vi "Lab Panel V5.31.vi"() -> ()   [LabVIEW 2017] (continued)
                            n2531 = Build Array(w4626) -> (w4623:dbl[])
                            n2532 = Build Array(w4631) -> (w4618:dbl[])
                            n2533 = Build Array("AMPS ON", "AMPS OFF", "VOLTS", "PF", "TEMP Live", "TEMP Neut", "CYCLE") -> (w4601:string[])
                            n2534 = Bundle By Name("Y"=w4624, "t0"=w4617) -> (w4616:waveform(dbl))  [unwired: 1 in]
                            n2535 = Bundle By Name("Y"=w4623, "t0"=w4617) -> (w4615:waveform(dbl))  [unwired: 1 in]
                            n2536 = Bundle By Name("Y"=w4622, "t0"=w4617) -> (w4614:waveform(dbl))  [unwired: 1 in]
                            n2537 = Bundle By Name("Y"=w4621, "t0"=w4617) -> (w4613:waveform(dbl))  [unwired: 1 in]
                            n2538 = Bundle By Name("Y"=w4620, "t0"=w4617) -> (w4612:waveform(dbl))  [unwired: 1 in]
                            n2539 = Bundle By Name("Y"=w4619, "t0"=w4617) -> (w4611:waveform(dbl))  [unwired: 1 in]
                            n2540 = Bundle By Name("Y"=w4618, "t0"=w4617) -> (w4610:waveform(dbl))  [unwired: 1 in]
                            n2541 = Build Array(w4616, w4615, w4614, w4613, w4612, w4611, w4610) -> (w4609:waveform(dbl)[])
                            n2542 = TDMS Write(0:w4630, 5:"TEST VALUES", 7:w4601, 9:w4609) -> (4:w4600:refnum<k34>, 6:w4599:string, 15:w4598:errorcluster)  [unwired: 2 in, 1 out]
                            n2543 = TDMS Write(0:w4600, 5:w4599, 7:"TIME", 9:w4596, 11:w4598) -> (15:w4595:errorcluster)  [unwired: 1 in, 3 out]
                            n2544 = local write "data file error"(w4595) -> ()
                          }
                        }
                      }
                    }
                  }
                }
              }
              frame #8 {
                n2545 = case shown="True" w4634 {
                  tunnel: w4638 -> [_ w4643]
                  tunnel: w4637 -> [_ w4642]
                  tunnel: w4636 -> [_ w4640]
                  tunnel: w4635 -> [_ w4639]
                  frame False {
                  }
                  frame True {
                    n2546 = local read "DISP LAB05-1"() -> (w4644:T4)
                    n2547 = local read "SIG LAB05-1"() -> (w4645:T2)
                    n2548 = local read "ON L05-1"() -> (w4641:cluster{"amps":dbl, "volts":dbl, "pf":dbl})
                    n2549 = Unbundle(w4645) -> ("AMPS"=w4651:dbl, "VOLTS"=w4649:dbl, "PF"=w4648:dbl, "Tmp Live"=w4647:dbl, "Tmp Neut"=w4650:dbl)
                    n2550 = Unbundle(w4644) -> ("CYCLE"=w4646:dbl)  [unwired: 2 out]
                    n2551 = stacked-sequence {
                      tunnel: w4651 -> [w4655 w4674]
                      tunnel: w4650 -> [_ w4673]
                      tunnel: w4649 -> [w4654 w4672]
                      tunnel: w4648 -> [w4653 w4671]
                      tunnel: w4647 -> [_ w4670]
                      tunnel: w4646 -> [_ w4669]
                      tunnel: w4643 -> [_ w4668]
                      tunnel: w4642 -> [w4656 _]
                      tunnel: w4641 -> [w4652 w4666]
                      tunnel: w4640 -> [_ w4667]
                      tunnel: w4639 -> [_ w4662]
                      frame #0 {
                        n2552 = case shown="True" w4656 {
                          tunnel: w4655 -> [_ w4661]
                          tunnel: w4654 -> [_ w4660]
                          tunnel: w4653 -> [_ w4659]
                          tunnel: w4652 -> [_ w4657]
                          frame False {
                          }
                          frame True {
                            n2553 = Bundle(cluster=w4657, "amps"=w4661, "volts"=w4660, "pf"=w4659) -> (w4658:cluster{"amps":dbl, "volts":dbl, "pf":dbl})
                            n2554 = local write "ON L05-1"(w4658) -> ()
                          }
                        }
                      }
                      frame #1 {
                        n2555 = Unbundle(w4666) -> ("amps"=w4665:dbl, "volts"=w4664:dbl, "pf"=w4663:dbl)
                        n2556 = case shown="True" w4667 {
                          tunnel: w4674 -> [_ w4706]
                          tunnel: w4673 -> [_ w4713]
                          tunnel: w4672 -> [_ _]
                          tunnel: w4671 -> [_ _]
                          tunnel: w4670 -> [_ w4712]
                          tunnel: w4669 -> [_ w4711]
                          tunnel: w4668 -> [_ w4676]
                          tunnel: w4665 -> [_ w4708]
                          tunnel: w4664 -> [_ w4707]
                          tunnel: w4663 -> [_ w4705]
                          tunnel: w4662 -> [_ w4697]
                          frame False {
                          }
                          frame True {
                            n2557 = local read "TDMS LAB05-1"() -> (w4710:refnum<k34>)
                            n2558 = Build Array(w4707) -> (w4702:dbl[])
                            n2559 = Build Array(w4705) -> (w4701:dbl[])
                            n2560 = Build Array(w4712) -> (w4700:dbl[])
                            n2561 = Build Array(w4713) -> (w4699:dbl[])
                            n2562 = Build Array(w4708) -> (w4704:dbl[])
                            n2563 = Build Array(w4706) -> (w4703:dbl[])
                            n2564 = Build Array(w4711) -> (w4698:dbl[])
                            n2565 = Build Array("AMPS ON", "AMPS OFF", "VOLTS", "PF", "TEMP Live", "TEMP Neut", "CYCLE") -> (w4681:string[])
                            n2566 = Bundle By Name("Y"=w4704, "t0"=w4697) -> (w4696:waveform(dbl))  [unwired: 1 in]
                            n2567 = Bundle By Name("Y"=w4703, "t0"=w4697) -> (w4695:waveform(dbl))  [unwired: 1 in]
                            n2568 = Bundle By Name("Y"=w4702, "t0"=w4697) -> (w4694:waveform(dbl))  [unwired: 1 in]
                            n2569 = Bundle By Name("Y"=w4701, "t0"=w4697) -> (w4693:waveform(dbl))  [unwired: 1 in]
                            n2570 = Bundle By Name("Y"=w4700, "t0"=w4697) -> (w4692:waveform(dbl))  [unwired: 1 in]
                            n2571 = Bundle By Name("Y"=w4699, "t0"=w4697) -> (w4691:waveform(dbl))  [unwired: 1 in]
                            n2572 = Bundle By Name("Y"=w4698, "t0"=w4697) -> (w4690:waveform(dbl))  [unwired: 1 in]
                            n2573 = Build Array(w4696, w4695, w4694, w4693, w4692, w4691, w4690) -> (w4689:waveform(dbl)[])
                            n2574 = TDMS Write(0:w4710, 5:"TEST VALUES", 7:w4681, 9:w4689) -> (4:w4680:refnum<k34>, 6:w4679:string, 15:w4678:errorcluster)  [unwired: 2 in, 1 out]
                            n2575 = TDMS Write(0:w4680, 5:w4679, 7:"TIME", 9:w4676, 11:w4678) -> (15:w4675:errorcluster)  [unwired: 1 in, 3 out]
                            n2576 = local write "data file error"(w4675) -> ()
                          }
                        }
                      }
                    }
                  }
                }
              }
              frame #9 {
                n2577 = case shown="True" w4714 {
                  tunnel: w4718 -> [_ w4723]
                  tunnel: w4717 -> [_ w4722]
                  tunnel: w4716 -> [_ w4720]
                  tunnel: w4715 -> [_ w4719]
                  frame False {
                  }
                  frame True {
                    n2578 = local read "DISP LAB05-2"() -> (w4724:T4)
                    n2579 = local read "SIG LAB05-2"() -> (w4725:T2)
                    n2580 = local read "ON L05-2"() -> (w4721:cluster{"amps":dbl, "volts":dbl, "pf":dbl})
                    n2581 = Unbundle(w4725) -> ("AMPS"=w4731:dbl, "VOLTS"=w4729:dbl, "PF"=w4728:dbl, "Tmp Live"=w4727:dbl, "Tmp Neut"=w4730:dbl)
                    n2582 = Unbundle(w4724) -> ("CYCLE"=w4726:dbl)  [unwired: 2 out]
                    n2583 = stacked-sequence {
                      tunnel: w4731 -> [w4735 w4754]
                      tunnel: w4730 -> [_ w4753]
                      tunnel: w4729 -> [w4734 w4752]
                      tunnel: w4728 -> [w4733 w4751]
                      tunnel: w4727 -> [_ w4750]
                      tunnel: w4726 -> [_ w4749]
                      tunnel: w4723 -> [_ w4748]
                      tunnel: w4722 -> [w4736 _]
                      tunnel: w4721 -> [w4732 w4746]
                      tunnel: w4720 -> [_ w4747]
                      tunnel: w4719 -> [_ w4742]
                      frame #0 {
                        n2584 = case shown="True" w4736 {
                          tunnel: w4735 -> [_ w4741]
                          tunnel: w4734 -> [_ w4740]
                          tunnel: w4733 -> [_ w4739]
                          tunnel: w4732 -> [_ w4737]
                          frame False {
                          }
                          frame True {
                            n2585 = Bundle(cluster=w4737, "amps"=w4741, "volts"=w4740, "pf"=w4739) -> (w4738:cluster{"amps":dbl, "volts":dbl, "pf":dbl})
                            n2586 = local write "ON L05-2"(w4738) -> ()
                          }
                        }
                      }
                      frame #1 {
                        n2587 = Unbundle(w4746) -> ("amps"=w4745:dbl, "volts"=w4744:dbl, "pf"=w4743:dbl)
                        n2588 = case shown="True" w4747 {
                          tunnel: w4754 -> [_ w4786]
                          tunnel: w4753 -> [_ w4793]
                          tunnel: w4752 -> [_ _]
                          tunnel: w4751 -> [_ _]
                          tunnel: w4750 -> [_ w4792]
                          tunnel: w4749 -> [_ w4791]
                          tunnel: w4748 -> [_ w4756]
                          tunnel: w4745 -> [_ w4788]
                          tunnel: w4744 -> [_ w4787]
                          tunnel: w4743 -> [_ w4785]
                          tunnel: w4742 -> [_ w4777]
                          frame False {
                          }
                          frame True {
                            n2589 = local read "TDMS LAB05-2"() -> (w4790:refnum<k34>)
                            n2590 = Build Array(w4787) -> (w4782:dbl[])
                            n2591 = Build Array(w4785) -> (w4781:dbl[])
                            n2592 = Build Array(w4792) -> (w4780:dbl[])
                            n2593 = Build Array(w4793) -> (w4779:dbl[])
                            n2594 = Build Array(w4788) -> (w4784:dbl[])
                            n2595 = Build Array(w4786) -> (w4783:dbl[])
                            n2596 = Build Array(w4791) -> (w4778:dbl[])
                            n2597 = Build Array("AMPS ON", "AMPS OFF", "VOLTS", "PF", "TEMP Live", "TEMP Neut", "CYCLE") -> (w4761:string[])
                            n2598 = Bundle By Name("Y"=w4784, "t0"=w4777) -> (w4776:waveform(dbl))  [unwired: 1 in]
                            n2599 = Bundle By Name("Y"=w4783, "t0"=w4777) -> (w4775:waveform(dbl))  [unwired: 1 in]
                            n2600 = Bundle By Name("Y"=w4782, "t0"=w4777) -> (w4774:waveform(dbl))  [unwired: 1 in]
                            n2601 = Bundle By Name("Y"=w4781, "t0"=w4777) -> (w4773:waveform(dbl))  [unwired: 1 in]
                            n2602 = Bundle By Name("Y"=w4780, "t0"=w4777) -> (w4772:waveform(dbl))  [unwired: 1 in]
                            n2603 = Bundle By Name("Y"=w4779, "t0"=w4777) -> (w4771:waveform(dbl))  [unwired: 1 in]
                            n2604 = Bundle By Name("Y"=w4778, "t0"=w4777) -> (w4770:waveform(dbl))  [unwired: 1 in]
                            n2605 = Build Array(w4776, w4775, w4774, w4773, w4772, w4771, w4770) -> (w4769:waveform(dbl)[])
                            n2606 = TDMS Write(0:w4790, 5:"TEST VALUES", 7:w4761, 9:w4769) -> (4:w4760:refnum<k34>, 6:w4759:string, 15:w4758:errorcluster)  [unwired: 2 in, 1 out]
                            n2607 = TDMS Write(0:w4760, 5:w4759, 7:"TIME", 9:w4756, 11:w4758) -> (15:w4755:errorcluster)  [unwired: 1 in, 3 out]
                            n2608 = local write "data file error"(w4755) -> ()
                          }
                        }
                      }
                    }
                  }
                }
              }
            }
          }
          frame #15 {
            # "display test values on chart"
            n2609 = local read "jig cycle"() -> (w4798:dbl)
            n2610 = local read "on loops"() -> (w4800:dbl)
            n2611 = Add(x=w4800, y=4) -> (x+y=w4797:dbl)
            n2612 = Equal?(x=w4798, y=3) -> (x = y?=w4796:bool)
            n2613 = Equal?(x=w4798, y=w4797) -> (x = y?=w4795:bool)
            n2614 = Or(x=w4796, y=w4795) -> (x .or. y?=w4794:bool)
            "graph flag" <- w4794
            n2615 = global write "Global display 3.vi" "graph flag"(w4794) -> ()
            n2616 = case shown="True" w4794 {
              frame False {
              }
              frame True {
                n2617 = local read "SIG LAB05-1"() -> (w4843:T2)
                n2618 = local read "SIG LAB04-2"() -> (w4844:T2)
                n2619 = local read "SIG LAB05-2"() -> (w4842:T2)
                n2620 = local read "SIG LAB04-1"() -> (w4845:T2)
                n2621 = local read "SIG LAB01-1"() -> (w4851:T2)
                n2622 = local read "SIG LAB03-1"() -> (w4847:T2)
                n2623 = local read "SIG LAB03-2"() -> (w4846:T2)
                n2624 = local read "SIG LAB02-2"() -> (w4848:T2)
                n2625 = local read "SIG LAB02-1"() -> (w4849:T2)
                n2626 = local read "SIG LAB01-2"() -> (w4850:T2)
                n2627 = Unbundle By Name(w4851) -> ("AMPS"=w4841:dbl, "VOLTS"=w4831:dbl, "Tmp Live"=w4821:dbl, "Tmp Neut"=w4811:dbl)
                n2628 = Unbundle(w4844) -> ("AMPS"=w4834:dbl, "VOLTS"=w4824:dbl, "Tmp Live"=w4814:dbl, "Tmp Neut"=w4804:dbl)  [unwired: 1 out]
                n2629 = Unbundle(w4843) -> ("AMPS"=w4833:dbl, "VOLTS"=w4823:dbl, "Tmp Live"=w4813:dbl, "Tmp Neut"=w4803:dbl)  [unwired: 1 out]
                n2630 = Unbundle(w4842) -> ("AMPS"=w4832:dbl, "VOLTS"=w4822:dbl, "Tmp Live"=w4812:dbl, "Tmp Neut"=w4802:dbl)  [unwired: 1 out]
                n2631 = Unbundle(w4845) -> ("AMPS"=w4835:dbl, "VOLTS"=w4825:dbl, "Tmp Live"=w4815:dbl, "Tmp Neut"=w4805:dbl)  [unwired: 1 out]
                n2632 = Unbundle(w4846) -> ("AMPS"=w4836:dbl, "VOLTS"=w4826:dbl, "Tmp Live"=w4816:dbl, "Tmp Neut"=w4806:dbl)  [unwired: 1 out]
                n2633 = Unbundle(w4847) -> ("AMPS"=w4837:dbl, "VOLTS"=w4827:dbl, "Tmp Live"=w4817:dbl, "Tmp Neut"=w4807:dbl)  [unwired: 1 out]
                n2634 = Unbundle(w4848) -> ("AMPS"=w4838:dbl, "VOLTS"=w4828:dbl, "Tmp Live"=w4818:dbl, "Tmp Neut"=w4808:dbl)  [unwired: 1 out]
                n2635 = Unbundle(w4849) -> ("AMPS"=w4839:dbl, "VOLTS"=w4829:dbl, "Tmp Live"=w4819:dbl, "Tmp Neut"=w4809:dbl)  [unwired: 1 out]
                n2636 = Unbundle(w4850) -> ("AMPS"=w4840:dbl, "VOLTS"=w4830:dbl, "Tmp Live"=w4820:dbl, "Tmp Neut"=w4810:dbl)  [unwired: 1 out]
                n2637 = stacked-sequence {
                  tunnel: w4841 -> [w4883 _ _]
                  tunnel: w4840 -> [w4882 _ _]
                  tunnel: w4839 -> [w4873 _ _]
                  tunnel: w4838 -> [w4872 _ _]
                  tunnel: w4837 -> [w4862 _ _]
                  tunnel: w4836 -> [w4861 _ _]
                  tunnel: w4835 -> [_ w4906 _]
                  tunnel: w4834 -> [_ w4905 _]
                  tunnel: w4833 -> [_ w4895 _]
                  tunnel: w4832 -> [_ w4894 _]
                  tunnel: w4831 -> [w4880 _ _]
                  tunnel: w4830 -> [w4879 _ _]
                  tunnel: w4829 -> [w4870 _ _]
                  tunnel: w4828 -> [w4869 _ _]
                  tunnel: w4827 -> [w4860 _ _]
                  tunnel: w4826 -> [w4859 _ _]
                  tunnel: w4825 -> [_ w4904 _]
                  tunnel: w4824 -> [_ w4903 _]
                  tunnel: w4823 -> [_ w4893 _]
                  tunnel: w4822 -> [_ w4892 _]
                  tunnel: w4821 -> [w4877 _ _]
                  tunnel: w4820 -> [w4875 _ _]
                  tunnel: w4819 -> [w4866 _ _]
                  tunnel: w4818 -> [w4864 _ _]
                  tunnel: w4817 -> [w4858 _ _]
                  tunnel: w4816 -> [w4856 _ _]
                  tunnel: w4815 -> [_ w4902 _]
                  tunnel: w4814 -> [_ w4900 _]
                  tunnel: w4813 -> [_ w4891 _]
                  tunnel: w4812 -> [_ w4889 _]
                  tunnel: w4811 -> [w4876 _ _]
                  tunnel: w4810 -> [w4874 _ _]
                  tunnel: w4809 -> [w4865 _ _]
                  tunnel: w4808 -> [w4863 _ _]
                  tunnel: w4807 -> [w4857 _ _]
                  tunnel: w4806 -> [w4855 _ _]
                  tunnel: w4805 -> [_ w4901 _]
                  tunnel: w4804 -> [_ w4899 _]
                  tunnel: w4803 -> [_ w4890 _]
                  tunnel: w4802 -> [_ w4888 _]
                  frame #0 {
                    n2638 = Merge Signals(w4883, w4882) -> (→"LAB01 AMPS":dynamicdata)
                    n2639 = Merge Signals(w4880, w4879) -> (→"LAB01 VOLTS":dynamicdata)
                    n2640 = Merge Signals(w4860, w4859) -> (→"LAB03 VOLTS":dynamicdata)
                    n2641 = Merge Signals(w4877, w4876, w4875, w4874) -> (→"LAB01 deg C":dynamicdata)
                    n2642 = Merge Signals(w4873, w4872) -> (→"LAB02 AMPS":dynamicdata)
                    n2643 = Merge Signals(w4866, w4865, w4864, w4863) -> (→"LAB02 deg C":dynamicdata)
                    n2644 = Merge Signals(w4858, w4857, w4856, w4855) -> (→"LAB03 deg C":dynamicdata)
                    n2645 = Merge Signals(w4870, w4869) -> (→"LAB02 VOLTS":dynamicdata)
                    n2646 = Merge Signals(w4862, w4861) -> (→"LAB03 AMPS":dynamicdata)
                  }
                  frame #1 {
                    n2647 = Merge Signals(w4893, w4892) -> (→"LAB05 VOLTS":dynamicdata)
                    n2648 = Merge Signals(w4906, w4905) -> (→"LAB04 AMPS":dynamicdata)
                    n2649 = Merge Signals(w4895, w4894) -> (→"LAB05 AMPS":dynamicdata)
                    n2650 = Merge Signals(w4891, w4890, w4889, w4888) -> (→"LAB05 deg C":dynamicdata)
                    n2651 = Merge Signals(w4902, w4901, w4900, w4899) -> (→"LAB04 deg C":dynamicdata)
                    n2652 = Merge Signals(w4904, w4903) -> (→"LAB04 VOLTS":dynamicdata)
                  }
                  frame #2 {
                    n2653 = local read "LAB05 VOLTS"() -> (w4914:dynamicdata)
                    n2654 = local read "LAB04 VOLTS"() -> (w4915:dynamicdata)
                    n2655 = local read "LAB05 AMPS"() -> (w4920:dynamicdata)
                    n2656 = local read "LAB02 VOLTS"() -> (w4917:dynamicdata)
                    n2657 = local read "LAB03 VOLTS"() -> (w4916:dynamicdata)
                    n2658 = local read "LAB01 VOLTS"() -> (w4918:dynamicdata)
                    n2659 = local read "LAB04 AMPS"() -> (w4921:dynamicdata)
                    n2660 = local read "LAB03 AMPS"() -> (w4922:dynamicdata)
                    n2661 = local read "LAB03 deg C"() -> (w4910:dynamicdata)
                    n2662 = local read "LAB02 AMPS"() -> (w4923:dynamicdata)
                    n2663 = local read "LAB04 deg C"() -> (w4909:dynamicdata)
                    n2664 = local read "LAB05 deg C"() -> (w4908:dynamicdata)
                    n2665 = local read "LAB02 deg C"() -> (w4911:dynamicdata)
                    n2666 = local read "LAB01 deg C"() -> (w4912:dynamicdata)
                    n2667 = local read "LAB01 AMPS"() -> (w4924:dynamicdata)
                    n2668 = Merge Signals(w4912, w4911, w4910, w4909, w4908) -> (w4907:dynamicdata)
                    n2669 = Merge Signals(w4924, w4923, w4922, w4921, w4920) -> (w4919:dynamicdata)
                    n2670 = Merge Signals(w4918, w4917, w4916, w4915, w4914) -> (w4913:dynamicdata)
                    n2671 = global write "Global display 3.vi" "graph volts"(w4913) -> ()
                    n2672 = global write "Global display 3.vi" "graph deg C"(w4907) -> ()
                    n2673 = global write "Global display 3.vi" "graph amps"(w4919) -> ()
                  }
                }
              }
            }
          }
          frame #16 {
            # "check for amps fail"
            # "check for cycle test & temperature rise fail conditions"
            n2674 = local read "on loops"() -> (w4951:dbl)
            n2675 = local read "jig cycle"() -> (w4948:dbl)
            n2676 = Add(x=w4951, y=5.0) -> (x+y=w4949:dbl)
            n2677 = Equal?(x=w4948, y=w4949) -> (x = y?=w4944:bool)
            n2678 = local read "jig cycle"() -> (w4953:dbl)
            n2679 = Equal?(x=w4953, y=3.0) -> (x = y?=w4946:bool)
            n2680 = local read "Fail Loops"() -> (w4925:dbl)
            n2681 = stacked-sequence {
              tunnel: w4947 -> [w4956 _ _ _ _ _ _ _ _ _]
              tunnel: w4946 -> [w4957 w4977 w4997 w5017 w5037 w5057 w5077 w5097 w5117 w5137]
              tunnel: w4945 -> [w4954 _ _ _ _ _ _ _ _ _]
              tunnel: w4944 -> [w4955 w4976 w4996 w5016 w5036 w5056 w5076 w5096 w5116 w5136]
              tunnel: w4943 -> [_ w4975 _ _ _ _ _ _ _ _]
              tunnel: w4942 -> [_ w4974 _ _ _ _ _ _ _ _]
              tunnel: w4941 -> [_ _ w4995 _ _ _ _ _ _ _]
              tunnel: w4940 -> [_ _ w4994 _ _ _ _ _ _ _]
              tunnel: w4939 -> [_ _ _ w5015 _ _ _ _ _ _]
              tunnel: w4938 -> [_ _ _ w5014 _ _ _ _ _ _]
              tunnel: w4937 -> [_ _ _ _ w5035 _ _ _ _ _]
              tunnel: w4936 -> [_ _ _ _ w5034 _ _ _ _ _]
              tunnel: w4935 -> [_ _ _ _ _ w5055 _ _ _ _]
              tunnel: w4934 -> [_ _ _ _ _ w5054 _ _ _ _]
              tunnel: w4933 -> [_ _ _ _ _ _ w5075 _ _ _]
              tunnel: w4932 -> [_ _ _ _ _ _ w5074 _ _ _]
              tunnel: w4931 -> [_ _ _ _ _ _ _ w5095 _ _]
              tunnel: w4930 -> [_ _ _ _ _ _ _ w5094 _ _]
              tunnel: w4929 -> [_ _ _ _ _ _ _ _ w5115 _]
              tunnel: w4928 -> [_ _ _ _ _ _ _ _ w5114 _]
              tunnel: w4927 -> [_ _ _ _ _ _ _ _ _ w5135]
              tunnel: w4926 -> [_ _ _ _ _ _ _ _ _ w5134]
              frame #0 {
                # "LAB01-1"
                n2682 = case shown="True" w4954 {
                  tunnel: w4957 -> [_ w4970]
                  tunnel: w4956 -> [_ w4967]
                  tunnel: w4955 -> [_ w4966]
                  frame False {
                  }
                  frame True {
                    n2683 = local read "TEMP START LAB01-1"() -> (w4972:cluster{"TL":dbl, "TN":dbl})
                    n2684 = local read "RESULT LAB01-1"() -> (w4961:bool)
                    n2685 = local read "FAIL LAB01-1"() -> (w4964:cluster{"LO":dbl, "HI":dbl})
                    n2686 = local read "TDMS LAB01-1"() -> (w4971:refnum<k34>)
                    n2687 = local read "SET LAB01-1"() -> (w4968:T6)
                    n2688 = local read "DISP LAB01-1"() -> (w4969:T4)
                    n2689 = local read "SIG LAB01-1"() -> (w4973:T2)
                    n2690 = Bundle("FAIL LAB01-1"=w4964, "SIG LAB01-1"=w4973, "TEMP START LAB01-1"=w4972, "DISP LAB01-1"=w4969, "SET LAB01-1"=w4968, "TDMS LAB01-1"=w4971) -> (w4958:T36)  [unwired: 1 in]
                    n2691 = call "sub vi - cycle&temp fail v7.vi"("Amps Lo?"=w4970, "Input Cluster"=w4958, "SELECT"=w4967, "Amps Hi?"=w4966, "Result In"=w4961) -> ("(FAIL) out"=w4963:cluster{"FAIL LO":dbl, "FAIL HI":dbl}, "(DISP) out"=w4959:T4, "T-RISE"=w4960:cluster{"T-RISE (L)":dbl, "T-RISE (N)":dbl}, "Result Out"=w4962:bool, "file error"=w4965:errorcluster)  [unwired: 10 in]
                    n2692 = local write "TEMP RISE LAB01-1"(w4960) -> ()
                    n2693 = local write "FAIL LAB01-1"(w4963) -> ()
                    n2694 = local write "DISP LAB01-1"(w4959) -> ()
                    n2695 = local write "RESULT LAB01-1"(w4962) -> ()
                    n2696 = local write "data file error"(w4965) -> ()
                  }
                }
              }
              frame #1 {
                # "LAB01-2"
                n2697 = case shown="True" w4975 {
                  tunnel: w4977 -> [_ w4990]
                  tunnel: w4974 -> [_ w4987]
                  tunnel: w4976 -> [_ w4986]
                  frame False {
                  }
                  frame True {
                    n2698 = local read "TEMP START LAB01-2"() -> (w4992:cluster{"TL":dbl, "TN":dbl})
                    n2699 = local read "FAIL LAB01-2"() -> (w4983:cluster{"LO":dbl, "HI":dbl})
                    n2700 = local read "TDMS LAB01-2"() -> (w4991:refnum<k34>)
                    n2701 = local read "SET LAB01-2"() -> (w4988:T5)
                    n2702 = local read "DISP LAB01-2"() -> (w4989:T4)
                    n2703 = local read "RESULT LAB01-2"() -> (w4980:bool)
                    n2704 = local read "SIG LAB01-2"() -> (w4993:T2)
                    n2705 = Bundle("FAIL LAB01-2"=w4983, "SIG LAB01-2"=w4993, "TEMP START LAB01-2"=w4992, "DISP LAB01-2"=w4989, "SET LAB01-2"=w4988, "TDMS LAB01-2"=w4991) -> (w4978:T37)  [unwired: 1 in]
                    n2706 = call "sub vi - cycle&temp fail v7.vi"("Amps Lo?"=w4990, "Input Cluster"=w4978, "SELECT"=w4987, "Amps Hi?"=w4986, "Result In"=w4980) -> ("(FAIL) out"=w4982:cluster{"FAIL LO":dbl, "FAIL HI":dbl}, "(DISP) out"=w4985:T4, "T-RISE"=w4979:cluster{"T-RISE (L)":dbl, "T-RISE (N)":dbl}, "Result Out"=w4981:bool, "file error"=w4984:errorcluster)  [unwired: 10 in]
                    n2707 = local write "TEMP RISE LAB01-2"(w4979) -> ()
                    n2708 = local write "FAIL LAB01-2"(w4982) -> ()
                    n2709 = local write "DISP LAB01-2"(w4985) -> ()
                    n2710 = local write "RESULT LAB01-2"(w4981) -> ()
                    n2711 = local write "data file error"(w4984) -> ()
                  }
                }
              }
              frame #2 {
                # "LAB02-1"
                n2712 = case shown="True" w4995 {
                  tunnel: w4997 -> [_ w5010]
                  tunnel: w4994 -> [_ w5007]
                  tunnel: w4996 -> [_ w5006]
                  frame False {
                  }
                  frame True {
                    n2713 = local read "TEMP START LAB02-1"() -> (w5012:cluster{"TL":dbl, "TN":dbl})
                    n2714 = local read "FAIL LAB02-1"() -> (w5003:cluster{"LO":dbl, "HI":dbl})
                    n2715 = local read "TDMS LAB02-1"() -> (w5011:refnum<k34>)
                    n2716 = local read "SET LAB02-1"() -> (w5008:T5)
                    n2717 = local read "DISP LAB02-1"() -> (w5009:T4)
                    n2718 = local read "SIG LAB02-1"() -> (w5013:T2)
                    n2719 = local read "RESULT LAB02-1"() -> (w5000:bool)
                    n2720 = Bundle("FAIL LAB02-1"=w5003, "SIG LAB02-1"=w5013, "TEMP START LAB02-1"=w5012, "DISP LAB02-1"=w5009, "SET LAB02-1"=w5008, "TDMS LAB02-1"=w5011) -> (w4998:T38)  [unwired: 1 in]
                    n2721 = call "sub vi - cycle&temp fail v7.vi"("Amps Lo?"=w5010, "Input Cluster"=w4998, "SELECT"=w5007, "Amps Hi?"=w5006, "Result In"=w5000) -> ("(FAIL) out"=w5002:cluster{"FAIL LO":dbl, "FAIL HI":dbl}, "(DISP) out"=w5005:T4, "T-RISE"=w4999:cluster{"T-RISE (L)":dbl, "T-RISE (N)":dbl}, "Result Out"=w5001:bool, "file error"=w5004:errorcluster)  [unwired: 10 in]
                    n2722 = local write "TEMP RISE LAB02-1"(w4999) -> ()
                    n2723 = local write "FAIL LAB02-1"(w5002) -> ()
                    n2724 = local write "DISP LAB02-1"(w5005) -> ()
                    n2725 = local write "RESULT LAB02-1"(w5001) -> ()
                    n2726 = local write "data file error"(w5004) -> ()
                  }
                }
              }
              frame #3 {
                # "LAB02-2"
                n2727 = case shown="True" w5015 {
                  tunnel: w5017 -> [_ w5030]
                  tunnel: w5014 -> [_ w5027]
                  tunnel: w5016 -> [_ w5026]
                  frame False {
                  }
                  frame True {
                    n2728 = local read "TEMP START LAB02-2"() -> (w5032:cluster{"TL":dbl, "TN":dbl})
                    n2729 = local read "FAIL LAB02-2"() -> (w5023:cluster{"LO":dbl, "HI":dbl})
                    n2730 = local read "TDMS LAB02-2"() -> (w5031:refnum<k34>)
                    n2731 = local read "SET LAB02-2"() -> (w5028:T5)
                    n2732 = local read "DISP LAB02-2"() -> (w5029:T4)
                    n2733 = local read "SIG LAB02-2"() -> (w5033:T2)
                    n2734 = local read "RESULT LAB02-2"() -> (w5020:bool)
                    n2735 = Bundle("FAIL LAB02-2"=w5023, "SIG LAB02-2"=w5033, "TEMP START LAB02-2"=w5032, "DISP LAB02-2"=w5029, "SET LAB02-2"=w5028, "TDMS LAB02-2"=w5031) -> (w5018:T39)  [unwired: 1 in]
                    n2736 = call "sub vi - cycle&temp fail v7.vi"("Amps Lo?"=w5030, "Input Cluster"=w5018, "SELECT"=w5027, "Amps Hi?"=w5026, "Result In"=w5020) -> ("(FAIL) out"=w5022:cluster{"FAIL LO":dbl, "FAIL HI":dbl}, "(DISP) out"=w5025:T4, "T-RISE"=w5019:cluster{"T-RISE (L)":dbl, "T-RISE (N)":dbl}, "Result Out"=w5021:bool, "file error"=w5024:errorcluster)  [unwired: 10 in]
                    n2737 = local write "TEMP RISE LAB02-2"(w5019) -> ()
                    n2738 = local write "FAIL LAB02-2"(w5022) -> ()
                    n2739 = local write "DISP LAB02-2"(w5025) -> ()
                    n2740 = local write "RESULT LAB02-2"(w5021) -> ()
                    n2741 = local write "data file error"(w5024) -> ()
                  }
                }
              }
              frame #4 {
                # "LAB03-1"
                n2742 = case shown="True" w5035 {
                  tunnel: w5037 -> [_ w5050]
                  tunnel: w5034 -> [_ w5047]
                  tunnel: w5036 -> [_ w5046]
                  frame False {
                  }
                  frame True {
                    n2743 = local read "TEMP START LAB03-1"() -> (w5052:cluster{"TL":dbl, "TN":dbl})
                    n2744 = local read "FAIL LAB03-1"() -> (w5043:cluster{"LO":dbl, "HI":dbl})
                    n2745 = local read "TDMS LAB03-1"() -> (w5051:refnum<k34>)
                    n2746 = local read "SET LAB03-1"() -> (w5048:T5)
                    n2747 = local read "DISP LAB03-1"() -> (w5049:T4)
                    n2748 = local read "SIG LAB03-1"() -> (w5053:T2)
                    n2749 = local read "RESULT LAB03-1"() -> (w5040:bool)
                    n2750 = Bundle("FAIL LAB03-1"=w5043, "SIG LAB03-1"=w5053, "TEMP START LAB03-1"=w5052, "DISP LAB03-1"=w5049, "SET LAB03-1"=w5048, "TDMS LAB03-1"=w5051) -> (w5038:T40)  [unwired: 1 in]
                    n2751 = call "sub vi - cycle&temp fail v7.vi"("Amps Lo?"=w5050, "Input Cluster"=w5038, "SELECT"=w5047, "Amps Hi?"=w5046, "Result In"=w5040) -> ("(FAIL) out"=w5042:cluster{"FAIL LO":dbl, "FAIL HI":dbl}, "(DISP) out"=w5045:T4, "T-RISE"=w5039:cluster{"T-RISE (L)":dbl, "T-RISE (N)":dbl}, "Result Out"=w5041:bool, "file error"=w5044:errorcluster)  [unwired: 10 in]
                    n2752 = local write "TEMP RISE LAB03-1"(w5039) -> ()
                    n2753 = local write "FAIL LAB03-1"(w5042) -> ()
                    n2754 = local write "DISP LAB03-1"(w5045) -> ()
                    n2755 = local write "RESULT LAB03-1"(w5041) -> ()
                    n2756 = local write "data file error"(w5044) -> ()
                  }
                }
              }
              frame #5 {
                # "LAB03-2"
                n2757 = case shown="True" w5055 {
                  tunnel: w5057 -> [_ w5070]
                  tunnel: w5054 -> [_ w5067]
                  tunnel: w5056 -> [_ w5066]
                  frame False {
                  }
                  frame True {
                    n2758 = local read "TEMP START LAB03-2"() -> (w5072:cluster{"TL":dbl, "TN":dbl})
                    n2759 = local read "FAIL LAB03-2"() -> (w5063:cluster{"LO":dbl, "HI":dbl})
                    n2760 = local read "TDMS LAB03-2"() -> (w5071:refnum<k34>)
                    n2761 = local read "SET LAB03-2"() -> (w5068:T5)
                    n2762 = local read "DISP LAB03-2"() -> (w5069:T4)
                    n2763 = local read "RESULT LAB03-2"() -> (w5060:bool)
                    n2764 = local read "SIG LAB03-2"() -> (w5073:T2)
                    n2765 = Bundle("FAIL LAB03-2"=w5063, "SIG LAB03-2"=w5073, "TEMP START LAB03-2"=w5072, "DISP LAB03-2"=w5069, "SET LAB03-2"=w5068, "TDMS LAB03-2"=w5071) -> (w5058:T41)  [unwired: 1 in]
                    n2766 = call "sub vi - cycle&temp fail v7.vi"("Amps Lo?"=w5070, "Input Cluster"=w5058, "SELECT"=w5067, "Amps Hi?"=w5066, "Result In"=w5060) -> ("(FAIL) out"=w5062:cluster{"FAIL LO":dbl, "FAIL HI":dbl}, "(DISP) out"=w5065:T4, "T-RISE"=w5059:cluster{"T-RISE (L)":dbl, "T-RISE (N)":dbl}, "Result Out"=w5061:bool, "file error"=w5064:errorcluster)  [unwired: 10 in]
                    n2767 = local write "FAIL LAB03-2"(w5062) -> ()
                    n2768 = local write "TEMP RISE LAB03-2"(w5059) -> ()
                    n2769 = local write "DISP LAB03-2"(w5065) -> ()
                    n2770 = local write "RESULT LAB03-2"(w5061) -> ()
                    n2771 = local write "data file error"(w5064) -> ()
                  }
                }
              }
              frame #6 {
                # "LAB04-1"
                n2772 = case shown="True" w5075 {
                  tunnel: w5077 -> [_ w5090]
                  tunnel: w5074 -> [_ w5087]
                  tunnel: w5076 -> [_ w5086]
                  frame False {
                  }
                  frame True {
                    n2773 = local read "TEMP START LAB04-1"() -> (w5092:cluster{"TL":dbl, "TN":dbl})
                    n2774 = local read "FAIL LAB04-1"() -> (w5083:cluster{"LO":dbl, "HI":dbl})
                    n2775 = local read "TDMS LAB04-1"() -> (w5091:refnum<k34>)
                    n2776 = local read "SET LAB04-1"() -> (w5088:T5)
                    n2777 = local read "DISP LAB04-1"() -> (w5089:T4)
                    n2778 = local read "SIG LAB04-1"() -> (w5093:T2)
                    n2779 = local read "RESULT LAB04-1"() -> (w5080:bool)
                    n2780 = Bundle("FAIL LAB04-1"=w5083, "SIG LAB04-1"=w5093, "TEMP START LAB04-1"=w5092, "DISP LAB04-1"=w5089, "SET LAB04-1"=w5088, "TDMS LAB04-1"=w5091) -> (w5078:T42)  [unwired: 1 in]
                    n2781 = call "sub vi - cycle&temp fail v7.vi"("Amps Lo?"=w5090, "Input Cluster"=w5078, "SELECT"=w5087, "Amps Hi?"=w5086, "Result In"=w5080) -> ("(FAIL) out"=w5082:cluster{"FAIL LO":dbl, "FAIL HI":dbl}, "(DISP) out"=w5085:T4, "T-RISE"=w5079:cluster{"T-RISE (L)":dbl, "T-RISE (N)":dbl}, "Result Out"=w5081:bool, "file error"=w5084:errorcluster)  [unwired: 10 in]
                    n2782 = local write "TEMP RISE LAB04-1"(w5079) -> ()
                    n2783 = local write "FAIL LAB04-1"(w5082) -> ()
                    n2784 = local write "DISP LAB04-1"(w5085) -> ()
                    n2785 = local write "RESULT LAB04-1"(w5081) -> ()
                    n2786 = local write "data file error"(w5084) -> ()
                  }
                }
              }
              frame #7 {
                # "LAB04-2"
                n2787 = case shown="True" w5095 {
                  tunnel: w5097 -> [_ w5110]
                  tunnel: w5094 -> [_ w5107]
                  tunnel: w5096 -> [_ w5106]
                  frame False {
                  }
                  frame True {
                    n2788 = local read "TEMP START LAB04-2"() -> (w5112:cluster{"TL":dbl, "TN":dbl})
                    n2789 = local read "FAIL LAB04-2"() -> (w5103:cluster{"LO":dbl, "HI":dbl})
                    n2790 = local read "TDMS LAB04-2"() -> (w5111:refnum<k34>)
                    n2791 = local read "SET LAB04-2"() -> (w5108:T5)
                    n2792 = local read "DISP LAB04-2"() -> (w5109:T4)
                    n2793 = local read "SIG LAB04-2"() -> (w5113:T2)
                    n2794 = local read "RESULT LAB04-2"() -> (w5100:bool)
                    n2795 = Bundle("FAIL LAB04-2"=w5103, "SIG LAB04-2"=w5113, "TEMP START LAB04-2"=w5112, "DISP LAB04-2"=w5109, "SET LAB04-2"=w5108, "TDMS LAB04-2"=w5111) -> (w5098:T43)  [unwired: 1 in]
                    n2796 = call "sub vi - cycle&temp fail v7.vi"("Amps Lo?"=w5110, "Input Cluster"=w5098, "SELECT"=w5107, "Amps Hi?"=w5106, "Result In"=w5100) -> ("(FAIL) out"=w5102:cluster{"FAIL LO":dbl, "FAIL HI":dbl}, "(DISP) out"=w5105:T4, "T-RISE"=w5099:cluster{"T-RISE (L)":dbl, "T-RISE (N)":dbl}, "Result Out"=w5101:bool, "file error"=w5104:errorcluster)  [unwired: 10 in]
                    n2797 = local write "TEMP RISE LAB04-2"(w5099) -> ()
                    n2798 = local write "FAIL LAB04-2"(w5102) -> ()
                    n2799 = local write "DISP LAB04-2"(w5105) -> ()
                    n2800 = local write "RESULT LAB04-2"(w5101) -> ()
                    n2801 = local write "data file error"(w5104) -> ()
                  }
                }
              }
              frame #8 {
                # "LAB05-1"
                n2802 = case shown="True" w5115 {
                  tunnel: w5117 -> [_ w5130]
                  tunnel: w5114 -> [_ w5127]
                  tunnel: w5116 -> [_ w5126]
                  frame False {
                  }
                  frame True {
                    n2803 = local read "TEMP START LAB05-1"() -> (w5132:cluster{"TL":dbl, "TN":dbl})
                    n2804 = local read "FAIL LAB05-1"() -> (w5123:cluster{"LO":dbl, "HI":dbl})
                    n2805 = local read "TDMS LAB05-1"() -> (w5131:refnum<k34>)
                    n2806 = local read "SET LAB05-1"() -> (w5128:T5)
                    n2807 = local read "DISP LAB05-1"() -> (w5129:T4)
                    n2808 = local read "SIG LAB05-1"() -> (w5133:T2)
                    n2809 = local read "RESULT LAB05-1"() -> (w5120:bool)
                    n2810 = Bundle("FAIL LAB05-1"=w5123, "SIG LAB05-1"=w5133, "TEMP START LAB05-1"=w5132, "DISP LAB05-1"=w5129, "SET LAB05-1"=w5128, "TDMS LAB05-1"=w5131) -> (w5118:T44)  [unwired: 1 in]
                    n2811 = call "sub vi - cycle&temp fail v7.vi"("Amps Lo?"=w5130, "Input Cluster"=w5118, "SELECT"=w5127, "Amps Hi?"=w5126, "Result In"=w5120) -> ("(FAIL) out"=w5122:cluster{"FAIL LO":dbl, "FAIL HI":dbl}, "(DISP) out"=w5125:T4, "T-RISE"=w5119:cluster{"T-RISE (L)":dbl, "T-RISE (N)":dbl}, "Result Out"=w5121:bool, "file error"=w5124:errorcluster)  [unwired: 10 in]
                    n2812 = local write "TEMP RISE LAB05-1"(w5119) -> ()
                    n2813 = local write "FAIL LAB05-1"(w5122) -> ()
                    n2814 = local write "DISP LAB05-1"(w5125) -> ()
                    n2815 = local write "RESULT LAB05-1"(w5121) -> ()
                    n2816 = local write "data file error"(w5124) -> ()
                  }
                }
              }
              frame #9 {
                # "LAB05-2"
                n2817 = case shown="True" w5135 {
                  tunnel: w5137 -> [_ w5150]
                  tunnel: w5134 -> [_ w5147]
                  tunnel: w5136 -> [_ w5146]
                  frame False {
                  }
                  frame True {
                    n2818 = local read "TEMP START LAB05-2"() -> (w5152:cluster{"TL":dbl, "TN":dbl})
                    n2819 = local read "FAIL LAB05-2"() -> (w5143:cluster{"LO":dbl, "HI":dbl})
                    n2820 = local read "TDMS LAB05-2"() -> (w5151:refnum<k34>)
                    n2821 = local read "SET LAB05-2"() -> (w5148:T5)
                    n2822 = local read "DISP LAB05-2"() -> (w5149:T4)
                    n2823 = local read "SIG LAB05-2"() -> (w5153:T2)
                    n2824 = local read "RESULT LAB05-2"() -> (w5140:bool)
                    n2825 = Bundle("FAIL LAB05-2"=w5143, "SIG LAB05-2"=w5153, "TEMP START LAB05-2"=w5152, "DISP LAB05-2"=w5149, "SET LAB05-2"=w5148, "TDMS LAB05-2"=w5151) -> (w5138:T45)  [unwired: 1 in]
                    n2826 = call "sub vi - cycle&temp fail v7.vi"("Amps Lo?"=w5150, "Input Cluster"=w5138, "SELECT"=w5147, "Amps Hi?"=w5146, "Result In"=w5140) -> ("(FAIL) out"=w5142:cluster{"FAIL LO":dbl, "FAIL HI":dbl}, "(DISP) out"=w5145:T4, "T-RISE"=w5139:cluster{"T-RISE (L)":dbl, "T-RISE (N)":dbl}, "Result Out"=w5141:bool, "file error"=w5144:errorcluster)  [unwired: 10 in]
                    n2827 = local write "TEMP RISE LAB05-2"(w5139) -> ()
                    n2828 = local write "FAIL LAB05-2"(w5142) -> ()
                    n2829 = local write "DISP LAB05-2"(w5145) -> ()
                    n2830 = local write "RESULT LAB05-2"(w5141) -> ()
                    n2831 = local write "data file error"(w5144) -> ()
                  }
                }
              }
            }
            n2832 = global write "Global 1.vi" "fail count"(w4925) -> ()
          }
          frame #17 {
            # "run calibration routine"
            n2833 = local read "SET (cal)"() -> (w5154:bool)
            n2834 = case shown="True" w5154 {
              frame False {
              }
              frame True {
                n2835 = stacked-sequence {
                  seq-local: [w5155 _ _] -> [_ w5157 _]
                  frame #0 {
                    n2836 = call "CALIBRATION PASSWORD"() -> ("PASSWORD"=w5155:string)  [unwired: 17 in, 2 out]
                  }
                  frame #1 {
                    n2837 = Equal?(x=w5157, y="7777") -> (x = y?=w5156:bool)
                    n2838 = case shown="True" w5156 {
                      frame False {
                      }
                      frame True {
                        n2839 = stacked-sequence {
                          frame #0 {
                            n2840 = local read "SAMPLES"() -> (w5159:dbl)
                            n2841 = local read "AI Task2"() -> (w5160:dbl)
                            n2842 = local read "AI Task1"() -> (w5161:dbl)
                            n2843 = local read "AI Task0"() -> (w5162:dbl)
                            n2844 = local read "Temp Test Cal"() -> (w5163:dbl)
                            n2845 = call "sub vi - calibration v2.vi"("Samples"=w5159, "Task2"=w5160, "Task1"=w5161, "Task0"=w5162, "Temp Test Cal"=w5163) -> ()  [unwired: 7 in]
                          }
                          frame #1 {
                            n2846 = call "sub vi - get calibration values v1.vi"() -> ("TEMP REF CAL"=w5164:dbl, "LAB01 (CAL)"=w5169:T15, "LAB02 (CAL)"=w5168:T16, "LAB03 (CAL)"=w5167:T15, "LAB04 (CAL)"=w5166:T15, "calibration file error out"=w5170:errorcluster, "LAB05 (CAL)"=w5165:T15)  [unwired: 9 in]
                            n2847 = local write "TEMP REF cal"(w5164) -> ()
                            n2848 = local write "cal file error out"(w5170) -> ()
                            n2849 = local write "CAL LAB04"(w5166) -> ()
                            n2850 = local write "CAL LAB05"(w5165) -> ()
                            n2851 = local write "CAL LAB01"(w5169) -> ()
                            n2852 = local write "CAL LAB02"(w5168) -> ()
                            n2853 = local write "CAL LAB03"(w5167) -> ()
                          }
                        }
                      }
                    }
                  }
                  frame #2 {
                    n2854 = local write "SET (cal)"(FALSE) -> ()
                  }
                }
              }
            }
          }
          frame #18 {
            # "save certain settings to file"
            n2855 = String To Path(string="c:\\crabtree\\Set Up\\") -> (path=w5173:path)
            n2856 = Build Path(base path=w5173, name or relative path="settings.bin") -> (appended path=w5175:path)
            n2857 = Build Path(base path=w5173, name or relative path="mail.bin") -> (appended path=w5172:path)
            n2858 = Create Folder(path (use dialog)=w5173) -> (error out=w5178:errorcluster)  [unwired: 2 in, 2 out]
            n2859 = call <vilib>:"Clear Errors.vi"("error in (no error)"=w5178) -> ()  [unwired: 5 in, 2 out]
            n2860 = stacked-sequence {
              seq-local: [w5190 _] -> [_ w5203]
              tunnel: w5175 -> [_ w5204]
              tunnel: w5172 -> [_ w5202]
              frame #0 {
                n2861 = local read "C drive data root dir"() -> (w5189:path)
                n2862 = local read "Select COM port"() -> (w5186:refnum<visa-resource-name>)
                n2863 = local read "Network Directory"() -> (w5195:path)
                n2864 = local read "SET LAB05-2"() -> (w5194:T5)
                n2865 = local read "SET LAB05-1"() -> (w5193:T5)
                n2866 = local read "SET LAB04-2"() -> (w5192:T5)
                n2867 = local read "SET LAB03-2"() -> (w5196:T5)
                n2868 = local read "SET LAB04-1"() -> (w5191:T5)
                n2869 = local read "SET LAB03-1"() -> (w5197:T5)
                n2870 = local read "SET LAB02-2"() -> (w5198:T5)
                n2871 = local read "SET LAB02-1"() -> (w5199:T5)
                n2872 = local read "SET LAB01-2"() -> (w5200:T5)
                n2873 = local read "SET LAB01-1"() -> (w5201:T6)
                n2874 = local read "Temp Delay Lps"() -> (w5185:dbl)
                n2875 = local read "Amps Fail level"() -> (w5181:dbl)
                n2876 = local read "Temp Test Cal"() -> (w5182:dbl)
                n2877 = local read "Temp Value"() -> (w5184:dbl)
                n2878 = local read "Mail Test File To:"() -> (w5180:string)
                n2879 = local read "Fail Loops"() -> (w5183:dbl)
                n2880 = local read "Mail Test Fail"() -> (w5179:bool)
                n2881 = local read "RATE (Hz)"() -> (w5188:dbl)
                n2882 = local read "SAMPLES"() -> (w5187:dbl)
                n2883 = Bundle("SET LAB01-1"=w5201, "SET LAB01-2"=w5200, "SET LAB02-1"=w5199, "SET LAB02-2"=w5198, "SET LAB03-1"=w5197, "SET LAB03-2"=w5196, "SET LAB04-1"=w5191, "SET LAB04-2"=w5192, "SET LAB05-1"=w5193, "SET LAB05-2"=w5194, "Network Directory"=w5195, "C drive data root dir"=w5189, "RATE (Hz)"=w5188, "SAMPLES"=w5187, "Select COM port"=w5186, "Temp Delay Lps"=w5185, "Temp Value"=w5184, "Fail Loops"=w5183, "Temp Test Cal"=w5182, "Amps Fail level"=w5181, "Mail Test File To:"=w5180, "Mail Test Fail"=w5179) -> (w5190:T24)  [unwired: 1 in]
              }
              frame #1 {
                n2884 = event shown="[1] \"SET LAB01-1\", \"SET LAB01-2\", \"SET LAB02-1\", \"SET LAB02-2\", \"SET LAB03-1\", \"SET LAB03-2\", \"SET LAB04-1\", \"SET LAB04-2\", \"SET LAB05-1\", \"SET LAB05-2\", \"Network Directory\", \"C drive data root dir\", \"RATE (Hz)\", \"SAMPLES\", \"Select COM port\", \"Temp Delay Lps\", \"Temp Value\", \"Fail Loops\", \"Temp Test Cal\", \"Amps Fail level\", \"Mail Test File To:\", \"Mail Test Fail\": Value Change" {
                  selector: _ -> [_ _ _]
                  dyn-events: _ -> [_ _ _]
                  timeout: 10.0 -> [_ _ _]
                  tunnel: w5204 -> [_ w5206 _]
                  tunnel: w5203 -> [_ w5207 _]
                  tunnel: w5202 -> [_ _ w5218]
                  event Timeout {
                    n2885 = event-data() -> ()  [unwired: 1 in, 3 out]
                  }
                  event "SET LAB01-2", "SET LAB02-1", "SET LAB02-2", "SET LAB03-1", "SET LAB03-2", "SET LAB04-1", "SET LAB04-2", "SET LAB05-1", "SET LAB05-2", "Network Directory", "C drive data root dir", "RATE (Hz)", "SAMPLES", "Select COM port", "Temp Delay Lps", "Temp Value", "Fail Loops", "Temp Test Cal", "Amps Fail level", "Mail Test File To:", "Mail Test Fail": Value Change {
                    n2886 = event-data() -> ()  [unwired: 1 in, 6 out]
                    n2887 = Open/Create/Replace File(file path (use dialog)=w5206, operation (0:open)=T18."replace or create") -> (refnum out=w5212:refnum<file>, error out=w5211:errorcluster)  [unwired: 4 in, 1 out]
                    n2888 = Write to Binary File(file (use dialog)=w5212, data=w5207, error in=w5211) -> (refnum out=w5210:refnum<file>, error out=w5209:errorcluster)  [unwired: 3 in, 1 out]
                    n2889 = Close File(refnum=w5210, error in=w5209) -> (error out=w5208:errorcluster)  [unwired: 1 out]
                    n2890 = local write "data file error"(w5208) -> ()
                  }
                  event "MAIL SETTINGS.OUT SERVER ADDRESS", "MAIL SETTINGS.FROM ACCOUNT", "MAIL SETTINGS.USER NAME", "MAIL SETTINGS.PASSWORD", "Auto Mail Send", "TO (string):": Value Change {
                    n2891 = event-data() -> ()  [unwired: 1 in, 6 out]
                    n2892 = local read "Auto Mail Send"() -> (w5215:bool)
                    n2893 = local read "MAIL SETTINGS"() -> (w5217:T8)
                    n2894 = local read "TO (string):"() -> (w5214:string)
                    n2895 = Open/Create/Replace File(file path (use dialog)=w5218, operation (0:open)=T18."replace or create") -> (refnum out=w5223:refnum<file>, error out=w5222:errorcluster)  [unwired: 4 in, 1 out]
                    n2896 = Bundle("MAIL SETTINGS"=w5217, "Auto Mail Send"=w5215, "TO (string):"=w5214) -> (w5216:T46)  [unwired: 1 in]
                    n2897 = Write to Binary File(file (use dialog)=w5223, data=w5216, error in=w5222) -> (refnum out=w5221:refnum<file>, error out=w5220:errorcluster)  [unwired: 3 in, 1 out]
                    n2898 = Close File(refnum=w5221, error in=w5220) -> (error out=w5219:errorcluster)  [unwired: 1 out]
                    n2899 = local write "data file error"(w5219) -> ()
                  }
                }
              }
            }
          }
          frame #19 {
            # "mail control"
            n2900 = local read "MAIL SETTINGS"() -> (w5240:T8)
            n2901 = local read "Auto Mail Send"() -> (w5226:bool)
            n2902 = Unbundle By Name(w5240) -> ("OUT SERVER ADDRESS"=w5239:string, "FROM ACCOUNT"=w5238:string, "TEST MAIL"=w5237:bool)
            n2903 = stacked-sequence {
              tunnel: "TO (string):" -> [_ w5279]
              tunnel: w5240 -> [w5245 w5278]
              tunnel: w5239 -> [w5244 w5277]
              tunnel: w5238 -> [w5243 w5276]
